vi "read_mcc_usb202.vi"(6 "error in":errorcluster, 11 "name":string="Dev1/Ai0:1") -> (0 "status":bool=TRUE, 3 "data":dbl[](array[numeric]), 4 "error out":errorcluster={"status"=TRUE, "code"=10023, "source"="ULx Create Channel (AI-Voltage-Basic).vi:5780001<ERR>\nMeasurements: Channel not specified."})   [LabVIEW 2019]
uses:
  <vilib>/ULx/Create Channel.llb/ULx Create Channel (AI-Voltage-Basic).vi
  <vilib>/ULx/Timing.llb/ULx Timing (Sample Clock).vi
  <vilib>/ULx/Read.llb/ULx Read (Analog 1D DBL NChan 1Samp).vi
panel:
  in  "Refnum":refnum<k21>
  # "\"Refnum\" is used only to find available devices."
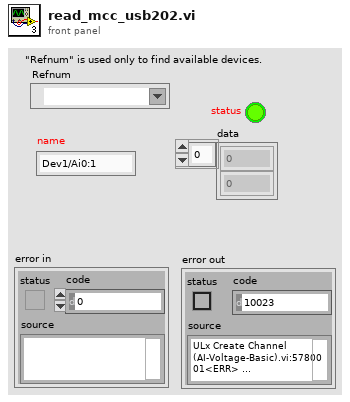
[diagram p1: front panel]
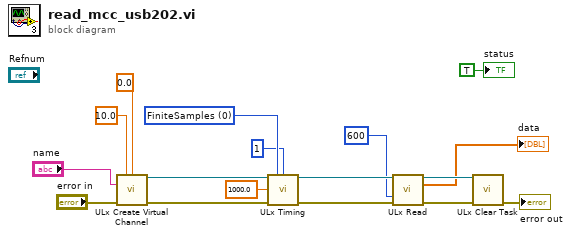
[diagram p0: block diagram]
diagram:
  w7 = 0 items=["FiniteSamples", "ContinuousSamples"] ("Sampling Mode")
  n1 = call-poly <vilib>:"ULx Create Virtual Channel.vi"("maximum value"=10.0 ("Max Value"), "minimum value"=0.0 ("Min Value"), "physical channels"="name", "error in"="error in") -> ("task out"=w11:refnum<k24>, "error out"=w12:errorcluster)  [unwired: 10 in]
  n2 = call-poly <vilib>:"ULx Timing.vi"("task in"=w11, "sample mode"=w7, "samples per channel"=1, "rate"=1000.0, "error in"=w12) -> ("task out"=w10:refnum<k24>, "error out"=w13:errorcluster)  [unwired: 9 in]
  n3 = call-poly <vilib>:"ULx Read.vi"("task in"=w10, "timeout"=600, "error in"=w13) -> ("task out"=w9:refnum<k24>, "data"=→"data":dbl[], "error out"=w8:errorcluster)  [unwired: 10 in]
  n4 = call <vilib>:"ULx Clear Task.vi"("task in"=w9, "error in"=w8) -> ("error out"=→"error out":errorcluster)  [unwired: 13 in]
  "status" <- TRUE ("status")
